vi "store_data.vi"(0 "abstract_datadestination_base in":refnum<class "abstract_datadestination_base.lvclass">, 5 "datas":refnum<class "abstract_data_base.lvclass">[](array[class]), 11 "error in (no error)":errorcluster) -> (4 "abstract_datadestination_base out":refnum<class "abstract_datadestination_base.lvclass">, 15 "error out":errorcluster)   [LabVIEW 2020, in "abstract_datadestination_base.lvclass"]
uses:
  abstract_datadestination_base.lvclass
  data/abstract_data_base/abstract_data_base.lvclass
  data/data_document/data_document.lvclass
  D:/Personal/LabVIEW LLMs/src/data/abstract_data_base/abstract_data_base.lvclass
  data/data_node/data_node.lvclass
  79a81340-23da-4116-af83-7f4da2d55596.vi
  <vilib>/Comparison/Equal/Equal Functor/Equal Functor.lvclass
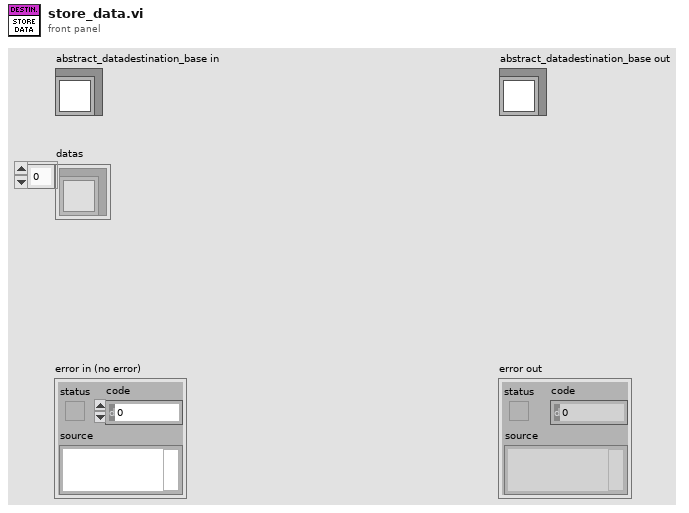
[diagram p1: front panel]
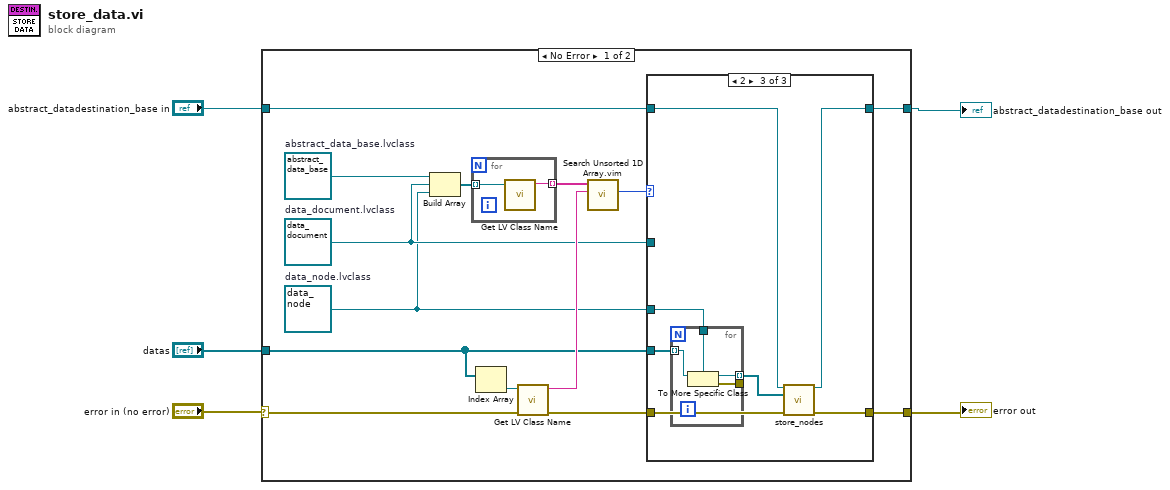
[diagram p0: block diagram]
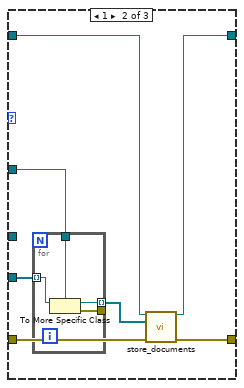
[diagram p3: hidden frame]
diagram:
  n1 = case shown="No Error" "error in (no error)" {
    selector: "error in (no error)" -> [w19 w47]
    tunnel: [w11 w47] -> w4
    tunnel: [w9 w46] -> w2
    tunnel: "abstract_datadestination_base in" -> [w10 w46]
    tunnel: "datas" -> [w8 _]
    frame No Error {
      w6 = refnum<class "data_node.lvclass"> refnum  # data_node.lvclass
      w7 = refnum<class "data_document.lvclass"> refnum  # data_document.lvclass
      w17 = refnum<class "abstract_data_base.lvclass"> refnum  # abstract_data_base.lvclass
      n2 = Build Array(w17, w7, w6) -> (w16:refnum<class "abstract_data_base.lvclass">[])
      n3 = for {
        tunnel: w16 -> [w45] mode=indexing
        tunnel: [w44] -> w15 mode=indexing
        n4 = call <vilib>:"Get LV Class Name.vi"("object"=w45) -> ("class name"=w44:string)  [unwired: 9 in, 1 out]
      }
      n5 = Index Array(array=w8) -> (element=w18:refnum<class "abstract_data_base.lvclass">)  [unwired: 1 in]
      n6 = call <vilib>:"Get LV Class Name.vi"("error in (no error)"=w19, "object"=w18) -> ("error out"=w13:errorcluster, "class name"=w14:string)  [unwired: 8 in]
      n7 = call "Search Unsorted 1D Array.vim"("element"=w14, "unsorted 1D array"=w15) -> ("index of element"=w12:i32)  [unwired: 9 in]
      n8 = case shown="2" w12 {
        tunnel: w13 -> [w21 w28 w39]
        tunnel: [w21 w27 w38] -> w11
        tunnel: w10 -> [w20 w26 w37]
        tunnel: [w20 w25 w36] -> w9
        tunnel: w8 -> [_ w24 w35]
        tunnel: w7 -> [_ w23 _]
        tunnel: w6 -> [_ _ w33]
        frame 0, Default {
        }
        frame 1 {
          n9 = for {
            tunnel: w24 -> [w32] mode=indexing
            tunnel: w23 -> [w31]
            tunnel: [w30] -> w22 mode=indexing
            tunnel: [w29] -> _
            n10 = To More Specific Class(target class=w31, reference=w32) -> (specific class reference=w30:refnum<class "data_document.lvclass">, error out=w29:errorcluster)  [unwired: 1 in]
          }
          n11 = call-dynamic "store_documents.vi"("abstract_datadestination_base in"=w26, "documents"=w22, "error in (no error)"=w28) -> ("abstract_datadestination_base out"=w25:refnum<class "abstract_datadestination_base.lvclass">, "error out"=w27:errorcluster)  [unwired: 11 in]
        }
        frame 2 {
          n12 = for {
            tunnel: w35 -> [w43] mode=indexing
            tunnel: w33 -> [w42]
            tunnel: [w41] -> w34 mode=indexing
            tunnel: [w40] -> _
            n13 = To More Specific Class(target class=w42, reference=w43) -> (specific class reference=w41:refnum<class "data_node.lvclass">, error out=w40:errorcluster)  [unwired: 1 in]
          }
          n14 = call-dynamic "store_nodes.vi"("abstract_datadestination_base in"=w37, "nodes"=w34, "error in (no error)"=w39) -> ("abstract_datadestination_base out"=w36:refnum<class "abstract_datadestination_base.lvclass">, "error out"=w38:errorcluster)  [unwired: 11 in]
        }
      }
    }
    frame Error {
    }
  }
  "error out" <- w4
  "abstract_datadestination_base out" <- w2
